vi "Find First Matching Resource (U32).vi"(6 "Error if not found? (F)":bool, 8 "error in (no error)":errorcluster, 10 "Resource Types":u32[](array[numeric]), 11 "Resources":T1[](array[typedef])) -> (0 "error out":errorcluster, 1 "Index":i32, 2 "Resource":T1, 3 "Resources out":T1[](array[typedef]), 5 "Found?":bool)   [LabVIEW 2026, in "VILab.lvlib"]
uses:
  VILab.lvlib
  CTLs/Resource.ctl
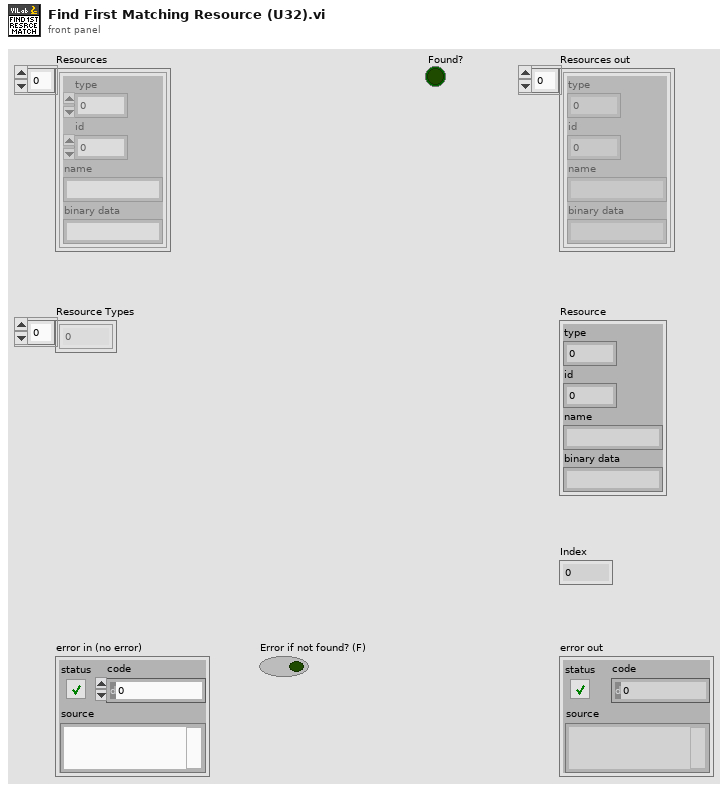
[diagram p1: front panel]
types:
  T1 = typedef "VILab.lvlib/Resource.ctl" = cluster{"type":u32, "id":i32, "name":string, "binary data":string}
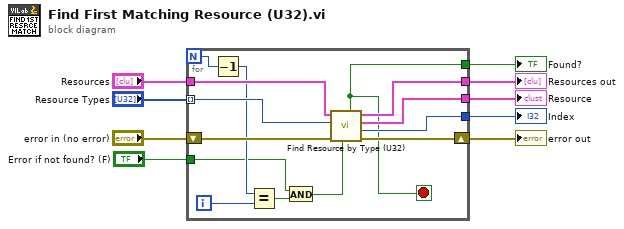
[diagram p0: block diagram]
diagram:
  n1 = for {
    N -> [w14]
    tunnel: "Resource Types" -> [w23] mode=indexing
    tunnel: "Resources" -> [w22]
    shift-right: [w20] -> w7
    shift-left: "error in (no error)" -> [w21]
    tunnel: [w11] -> w3
    tunnel: "Error if not found? (F)" -> [w16]
    tunnel: [w13] -> w4
    tunnel: [w12] -> w2
    tunnel: [w10] -> w1
    i -> [w18]
    stop <- w10 stop-if-true
    n2 = Decrement(x=w14) -> (x-1=w19:i32)
    n3 = Equal?(x=w19, y=w18) -> (x = y?=w17:bool)
    n4 = And(x=w16, y=w17) -> (x .and. y?=w15:bool)
    n5 = call "Find Resource by Type (U32).vi"("Error if not found? (F)"=w15, "error in (no error)"=w21, "Resource Type"=w23, "Resources"=w22) -> ("error out"=w20:errorcluster, "Index"=w13:i32, "Resource"=w12:T1, "Resources out"=w11:T1[], "Found?"=w10:bool)  [unwired: 3 in]
  }
  "error out" <- w7
  "Index" <- w4
  "Resource" <- w2
  "Found?" <- w1
  "Resources out" <- w3
